vi "Get Headers.vi"(8 "error in (no error)":errorcluster, 11 "HttpContent in":refnum<class "HttpContent.lvclass">) -> (0 "error out":errorcluster, 2 "HTTPHeaders":refnum<class "HttpHeaders_Content.lvclass">, 3 "HttpContent out":refnum<class "HttpContent.lvclass">)   [LabVIEW 2018, in "HttpClient_NET.lvlib" / "HttpContent.lvclass"]
doc: "<b> </b> <b> </b>\nHttpClient_NET\nJustin Young - Viviota\nCopyright (c) 2021\nLicense: BSD"
uses:
  HttpContent.lvclass
  HttpHeaders_content/HttpHeaders_Content.lvclass
  C:/Viviota/Projects/R&D/__OpenSource/VIV_HTTP_REST_NET/HTTPHeaders_NET/HttpHeaders_NET.lvclass
  HttpContent.lvclass/HttpContent.ctl
  Accessors/Read NET_HttpContent.vi
  System.Net.Http
  HTTPHeaders_NET/HttpHeaders_NET.lvclass
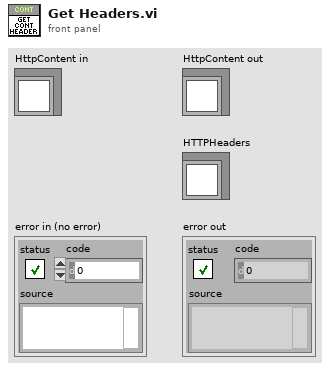
[diagram p1: front panel]
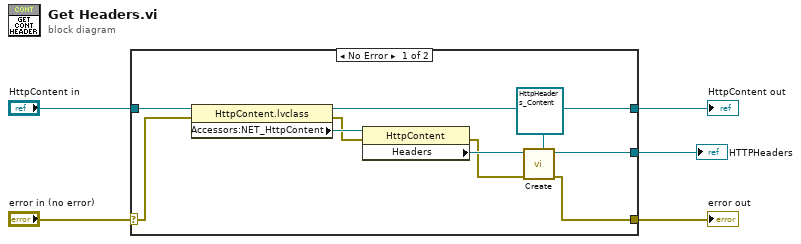
[diagram p0: block diagram]
diagram:
  n1 = case shown="No Error" "error in (no error)" {
    selector: "error in (no error)" -> [w9 w17]
    tunnel: [w6 w17] -> w4
    tunnel: [w14 w16] -> w2
    tunnel: "HttpContent in" -> [w15 w16]
    tunnel: [w10 _] -> w1
    frame No Error {
      n2 = property class="HttpContent.lvclass"(reference=w15, error in=w9) -> (reference out=w14:refnum<class "HttpContent.lvclass">, error out=w8:errorcluster, "Accessors:NET_HttpContent"=w13:refnum<k24>)
      n3 = property class="HttpContent"(reference=w13, error in=w8) -> (error out=w7:errorcluster, "Headers"=w12:refnum<k24>)  [unwired: 1 out]
      n4 = call "Create.vi"("HTTPHeaders_NET in"=refnum<class "HttpHeaders_Content.lvclass"> refnum ("LabVIEWHTTPClient_NET.lvlib:HttpHeaders_Content"), "error in (no error)"=w7, "NET_HttpHeaders"=w12) -> ("error out"=w6:errorcluster, "HTTPHeaders_NET out"=w10:refnum<class "HttpHeaders_Content.lvclass">)  [unwired: 7 in]
    }
    frame Error {
    }
  }
  "error out" <- w4
  "HttpContent out" <- w2
  "HTTPHeaders" <- w1
